vi "test-linear-system-loop-01.vi"() -> (3 "TEst Passed":bool)   [LabVIEW 2019]
uses:
  <vilib>/Rock Robotics/WPI/ThirdParty/JAS_Junk/TrajLib/Trajectory_Library.lvlib
  <vilib>/ptbypt/NI_PtbyPt.lvlib
  <vilib>/Rock Robotics/WPI/ThirdParty/JAS_Junk/TrajLib/DCMotor_GetVex775Pro.vi
  <vilib>/Analysis/Matrix/Datatypes/RealMatrix.ctl
  <vilib>/Analysis/Matrix/NI_Matrix.lvlib
  <vilib>/Rock Robotics/WPI/ThirdParty/JAS_Junk/TrajLib/TypeDef/LINEAR_QUADRATIC_REGULATOR.ctl
  <vilib>/Rock Robotics/WPI/ThirdParty/JAS_Junk/TrajLib/TypeDef/LINEAR_PLANT_INV_FF.ctl
  <vilib>/Rock Robotics/WPI/ThirdParty/JAS_Junk/TrajLib/TypeDef/LINEAR_SYSTEM.ctl
  <vilib>/Rock Robotics/WPI/ThirdParty/JAS_Junk/TrajLib/TypeDef/KALMAN_FILTER.ctl
  <vilib>/Rock Robotics/WPI/ThirdParty/JAS_Junk/TrajLib/TypeDef/LINEAR_SYSTEM_LOOP.ctl
panel:
  out "Waveform Graph":dbl[][](graph)
  out "Issue":bool
  out "Error":bool
  out "CorrError":bool
  out "out Linear System Loop":T1
  out "CalcYErr":bool
  out "LinSysLoopErr":bool
  out "LQRError":bool
  out "KalmanError":errorcluster
  out "Elev Sstem Err":bool
  # "<States,1>"
  # "<FUTURE --- CLAMP TYPE -- For now\nuse Normalize>"
  # "Steady State Gain  \n<States,Outputs>"
  # "State Estimate <Statess,1>"
  # "<States,States>"
  # "<States,Inputs>"
  # "<Outputs,States>"
  # "<Outputs,Inputs>"
  # "<States,1>"
  # "<Inputs,1>"
  # "<States,Inputs>"
  # "<States,States>"
  # "Ref State <States,1>"
  # "Comp and capped \noutput <Inputs,1>"
  # "Controller gain\n<Inputs,States>"
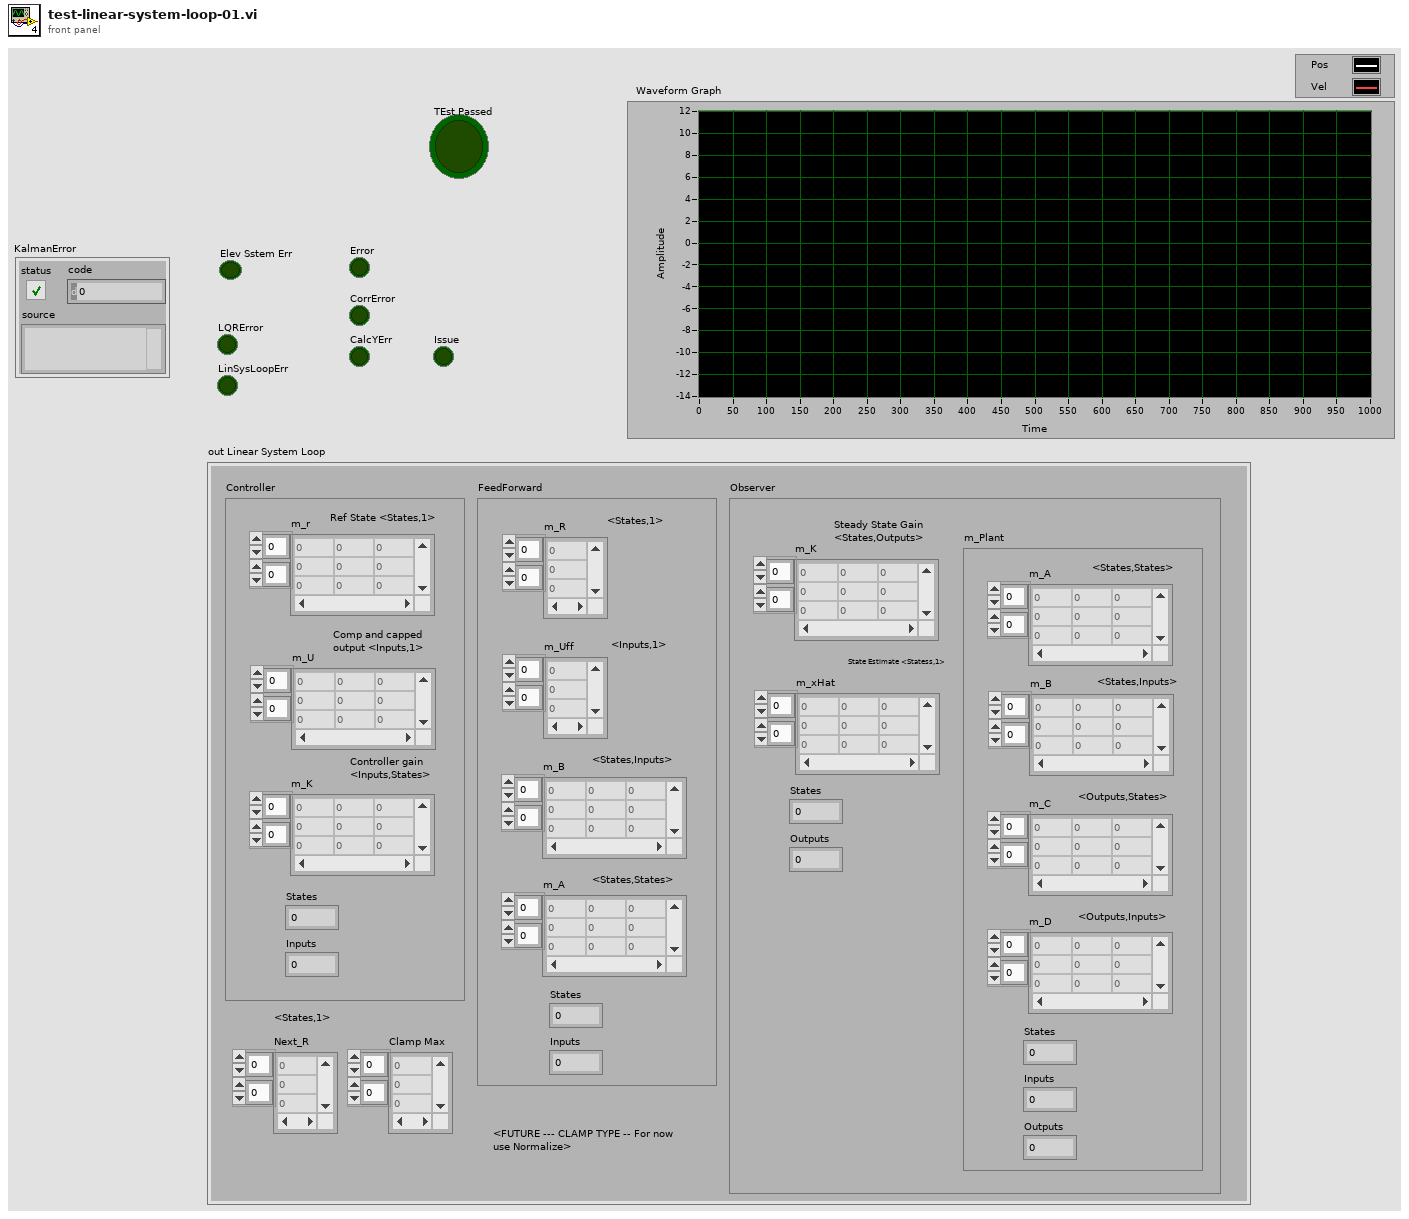
[diagram p1: front panel]
types:
  T1 = typedef "Trajectory_Library.lvlib/LINEAR_SYSTEM_LOOP.ctl" = cluster{"Controller":T2, "FeedForward":T4, "Observer":T5, "Next_R":T3, "Clamp Max":T3}
  T2 = typedef "Trajectory_Library.lvlib/LINEAR_QUADRATIC_REGULATOR.ctl" = cluster{"m_r":T3, "m_U":T3, "m_K":T3, "States":i32, "Inputs":i32}
  T3 = typedef "NI_Matrix.lvlib/RealMatrix.ctl" = dbl[][]
  T4 = typedef "Trajectory_Library.lvlib/LINEAR_PLANT_INV_FF.ctl" = cluster{"m_R":T3, "m_Uff":T3, "m_B":T3, "m_A":T3, "States":i32, "Inputs":i32}
  T5 = typedef "Trajectory_Library.lvlib/KALMAN_FILTER.ctl" = cluster{"m_K":T3, "m_xHat":T3, "States":i32, "Outputs":i32, "m_Plant":T6}
  T6 = typedef "Trajectory_Library.lvlib/LINEAR_SYSTEM.ctl" = cluster{"m_A":T3, "m_B":T3, "m_C":T3, "m_D":T3, "States":i32, "Inputs":i32, "Outputs":i32}
  T7 = typedef "Trajectory_Library.lvlib/DCMOTOR.CTL" = cluster{"nominalVoltage_Volts":dbl, "StallTorque_NM":dbl, "StallCurrent_Amps":dbl, "FreeCurrent_Amps":dbl, "FreeSpeed_RadPerSec":dbl, "R_Ohms":dbl, "KvINV_RadPerSecPerVolt":dbl, "Kt_NMPerAmp":dbl, "L_H":dbl, "Jr_KgM2":dbl}
  T8 = typedef "Trajectory_Library.lvlib/TRAPEZOID_PROFILE_CONSTRAINT.ctl" = cluster{"MaxVelocity":dbl, "MaxAcceleration":dbl}
  T9 = typedef "Trajectory_Library.lvlib/TRAPEZOID_PROFILE_STATE.ctl" = cluster{"Position":dbl, "Velocity":dbl}
  T10 = typedef "Trajectory_Library.lvlib/TRAPEZOID_PROFILE.ctl" = cluster{"EndAccel":dbl, "EndFullSpeed":dbl, "EndDecel":dbl, "Direction":i32, "Constraints":T8, "Initial":T9, "Goal":T9}
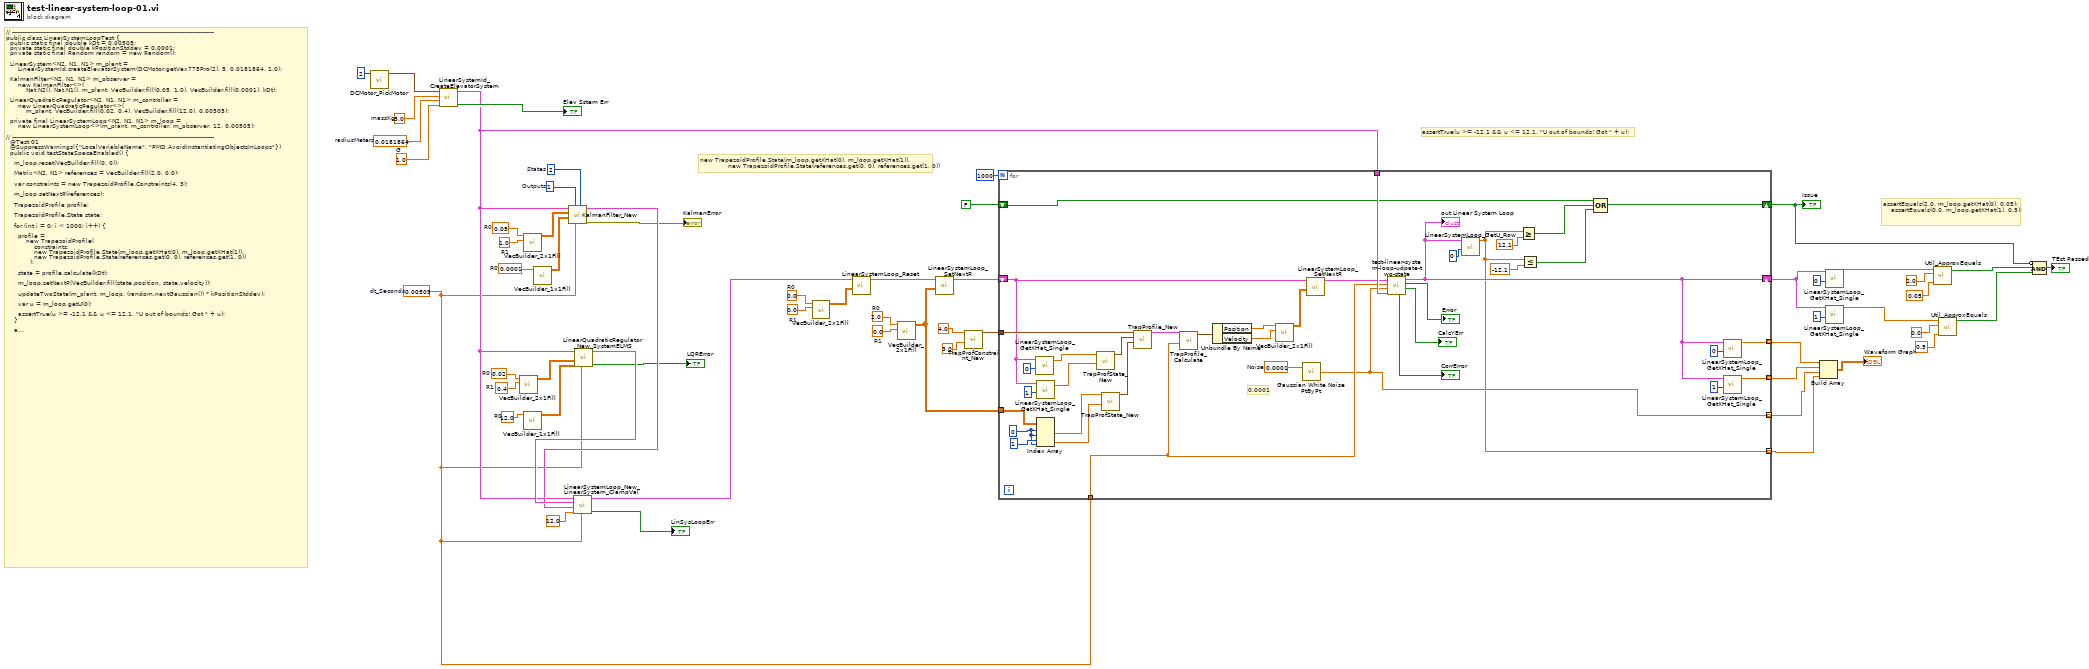
[diagram p0: block diagram]
diagram:
  w28 = 0.0  # R1
  w27 = 2.0  # R0
  w35 = 0.0  # R1
  w34 = 0.0  # R0
  w45 = 12.0  # R0
  w47 = 0.4  # R1
  w46 = 0.02  # R0
  w49 = 0.0001  # R0
  w51 = 1.0  # R1
  w50 = 0.05  # R0
  w52 = 1  # Outputs
  w21 = 0.00505  # dt_Seconds
  w53 = 2  # States
  w56 = 5.0  # massKg
  w57 = 0.0181864  # radiusMeters
  w58 = 1.0  # G
  # "assertEquals(2.0, m_loop.getXHat(0), 0.05);\n    assertEquals(0.0, m_loop.getXHat(1), 0.5);"
  # "assertTrue(u >= -12.1 && u <= 12.1, \"U out of bounds! Got \" + u);"
  # "new TrapezoidProfile.State(m_loop.getXHat(0), m_loop.getXHat(1)),\n              new TrapezoidProfile.State(references.get(0, 0), references.get(1, 0))"
  # "// -----------------------------------------------------------------------------------------------------\npublic class LinearSystemLoopTest {\n  public static final double kDt = 0.00505;\n  private static final double kPositionStddev = 0.0001;\n  private static final Random random = new Random();\n\n  LinearSystem<N2, N1, N1> m_plant =\n      LinearSystemId.createElevatorSystem(DCMotor.getVex775Pro(2), 5, 0.0181864, 1.0);\n\n  KalmanFilter<N2, N1, N1> m_observer =\n      new KalmanFilter<>(\n          Nat.N2(), Nat.N1(), m_plant, VecBuilder.fill(0.05, 1.0), VecBuilder.fill(0.0001), kDt);\n\n  LinearQuadraticRegulator<N2, N1, N1> m_controller =\n      new LinearQuadraticRegulator<>(\n          m_plant, VecBuilder.fill(0.02, 0.4), VecBuilder.fill(12.0), 0.00505);\n\n  private final LinearSystemLoop<N2, N1, N1> m_loop =\n      new LinearSystemLoop<>(m_plant, m_controller, m_observer, 12, 0.00505);\n\n// -----------------------------------------------------------------------------------------------------\n  @Test 01\n  @SuppressWarnings({\"LocalVariableName\", \"PMD.AvoidInstantiatingObjectsInLoops\"})\n  public void testStateSpaceEnabled() {\n\n    m_loop.reset(VecBuilder.fill(0, 0));\n\n    Matrix<N2, N1> references = VecBuilder.fill(2.0, 0.0);\n\n    var constraints = new TrapezoidProfile.Constraints(4, 3);\n\n    m_loop.setNextR(references);\n\n    TrapezoidProfile profile;\n\n    TrapezoidProfile.State state;\n\n    for (int i = 0; i < 1000; i++) {\n\n      profile =\n          new TrapezoidProfile(\n              constraints,\n              new TrapezoidProfile.State(m_loop.getXHat(0), m_loop.getXHat(1)),\n              new TrapezoidProfile.State(references.get(0, 0), references.get(1, 0))\n            );\n\n      state = profile.calculate(kDt);\n\n      m_loop.setNextR(VecBuilder.fill(state.position, state.velocity));\n\n      updateTwoState(m_plant, m_loop, (random.nextGaussian()) * kPositionStddev);\n\n      var u = m_loop.getU(0);\n\n      assertTrue(u >= -12.1 && u <= 12.1, \"U out of bounds! Got \" + u);\n    }\n\n    assertEquals(2.0, m_loop.getXHat(0), 0.05);\n    assertEquals(0.0, m_loop.getXHat(1), 0.5);\n  }"
  n1 = call-poly <vilib>:"DCMotor_PickMotor.vi"("Num Motors"=2) -> ("DCMOTOR"=w54:T7)  [unwired: 10 in]
  n2 = call <vilib>:"LinearSystemId_CreateElevatorSystem.vi"("G"=w58, "radiusMeters"=w57, "massKg"=w56, "DCMOTOR"=w54) -> ("Size Coerced"=→"Elev Sstem Err":bool, "Linearsystem"=w33:T6)  [unwired: 6 in]
  n3 = call <vilib>:"VecBuilder_2x1Fill.vi"("R1"=w47, "R0"=w46) -> ("output matrix"=w44:T3)  [unwired: 9 in]
  n4 = call <vilib>:"VecBuilder_1x1Fill.vi"("R0_C0"=w45) -> ("output matrix"=w43:T3)  [unwired: 10 in]
  n5 = call <vilib>:"VecBuilder_2x1Fill.vi"("R1"=w51, "R0"=w50) -> ("output matrix"=w48:T3)  [unwired: 9 in]
  n6 = call <vilib>:"VecBuilder_1x1Fill.vi"("R0_C0"=w49) -> ("output matrix"=w26:T3)  [unwired: 10 in]
  n7 = call <vilib>:"KalmanFilter_New.vi"("States"=w53, "dt_Seconds"=w21, "Outputs"=w52, "MeasurementStdDevs"=w26, "StateStdDevs"=w48, "Plant"=w33) -> ("Error"=→"KalmanError":errorcluster, "KalmanFilter"=w41:T5)  [unwired: 4 in]
  n8 = call <vilib>:"LinearQuadraticRegulator_New_SystemELMS.vi"("dt_Seconds"=w21, "Relms"=w43, "Qelms"=w44, "LINEARSYSTEM"=w33) -> ("Error"=→"LQRError":bool, "LinearQuadraticRegulator"=w42:T2)  [unwired: 6 in]
  n9 = call <vilib>:"LinearSystemLoop_New_LinearSystem_ClampVal.vi"("dT_Seconds"=w21, "Max_Voltage"=12.0, "Observer"=w41, "Controller"=w42, "Plant"=w33) -> ("Error"=→"LinSysLoopErr":bool, "Linear System Loop"=w32:T1)  [unwired: 5 in]
  n10 = call <vilib>:"VecBuilder_2x1Fill.vi"("R1"=w35, "R0"=w34) -> ("output matrix"=w31:T3)  [unwired: 9 in]
  n11 = call <vilib>:"LinearSystemLoop_Reset.vi"("initialState"=w31, "input inear System Loop"=w32) -> ("out Linear System Loop"=w30:T1)  [unwired: 8 in, 1 out]
  n12 = call <vilib>:"VecBuilder_2x1Fill.vi"("R1"=w28, "R0"=w27) -> ("output matrix"=w20:T3)  [unwired: 9 in]
  n13 = call <vilib>:"LinearSystemLoop_SetNextR.vi"("R"=w20, "input inear System Loop"=w30) -> ("out Linear System Loop"=w29:T1)  [unwired: 8 in, 1 out]
  n14 = call <vilib>:"TrapProfConstraint_New.vi"("Max Accel"=3.0, "Max Speed (M/S)"=4.0) -> ("TRAPEZOID_PROFILE_CONSTRAINT"=w22:T8)  [unwired: 9 in]
  n15 = for {
    N: 1000 -> [_]
    tunnel: w33 -> [w94]
    tunnel: w21 -> [w80]
    shift-right: [w63] -> w18
    shift-left: w29 -> [w76]
    tunnel: w22 -> [w93]
    tunnel: w20 -> [w84]
    shift-right: [w67] -> w6
    shift-left: FALSE -> [w66]
    tunnel: [w62] -> w9 mode=indexing
    tunnel: [w61] -> w8 mode=indexing
    tunnel: [w60] -> w2 mode=indexing
    tunnel: [w59] -> w1 mode=indexing
    w85 = 0 ("index (row)")
    w73 = 0.0001  # Noise
    # "0.0001"
    n16 = call <vilib>:"LinearSystemLoop_GetXHat_Single.vi"("Row"=0, "input inear System Loop"=w76) -> ("XHat"=w88:dbl)  [unwired: 9 in]
    n17 = call <vilib>:"LinearSystemLoop_GetXHat_Single.vi"("Row"=1, "input inear System Loop"=w76) -> ("XHat"=w87:dbl)  [unwired: 9 in]
    n18 = Index Array(array=w84, index (row) #1=w85, index (col) #1=w85, index (row) #2=1 ("index (row)"), index (col) #2=w85) -> (element #1=w83:dbl, element #2=w82:dbl)
    n19 = call <vilib>:"TrapProfState_New.vi"("Velocity"=w87, "Position"=w88) -> ("TRAPEZOID_PROFILE_STATE"=w92:T9)  [unwired: 9 in]
    n20 = call <vilib>:"TrapProfState_New.vi"("Velocity"=w82, "Position"=w83) -> ("TRAPEZOID_PROFILE_STATE"=w91:T9)  [unwired: 9 in]
    n21 = call <vilib>:"TrapProfile_New.vi"("Initial"=w91, "Goal"=w92, "Constraints"=w93) -> ("TRAPEZOID_PROFILE"=w81:T10)  [unwired: 8 in]
    n22 = call <vilib>:"TrapProfile_Calculate.vi"("Time"=w80, "TRAPEZOID_PROFILE"=w81) -> ("State"=w79:T9)  [unwired: 9 in]
    n23 = Unbundle By Name(w79) -> ("Position"=w78:dbl, "Velocity"=w77:dbl)
    n24 = call <vilib>:"VecBuilder_2x1Fill.vi"("R1"=w77, "R0"=w78) -> ("output matrix"=w74:T3)  [unwired: 9 in]
    n25 = call <vilib>:"Gaussian White Noise PtByPt.vi"("standard deviation"=w73) -> ("Gaussian white noise"=w60:dbl)  [unwired: 2 in]
    n26 = call <vilib>:"LinearSystemLoop_SetNextR.vi"("R"=w74, "input inear System Loop"=w76) -> ("out Linear System Loop"=w75:T1)  [unwired: 8 in, 1 out]
    n27 = call "test-linear-system-loop-udpate-two-state.vi"("Linearsystem"=w94, "Noise"=w60, "dt_Seconds"=w80, "Linear System Loop"=w75) -> ("CalcYErr"=→"CalcYErr":bool, "PredictError"=→"Error":bool, "out Linear System Loop"=w63:T1, "CorrectError"=→"CorrError":bool)  [unwired: 4 in]
    "out Linear System Loop" <- w63
    n28 = call <vilib>:"LinearSystemLoop_GetU_Row.vi"("Row"=0, "input inear System Loop"=w63) -> ("U"=w59:dbl)  [unwired: 9 in]
    n29 = Greater Or Equal?(x=w59, y=12.1) -> (x >= y?=w68:bool)
    n30 = Less Or Equal?(x=w59, y=-12.1) -> (x <= y?=w69:bool)
    n31 = Compound Arithmetic op=OR(w66, w68, w69) -> (w67:bool)
    n32 = call <vilib>:"LinearSystemLoop_GetXHat_Single.vi"("Row"=0, "input inear System Loop"=w63) -> ("XHat"=w62:dbl)  [unwired: 9 in]
    n33 = call <vilib>:"LinearSystemLoop_GetXHat_Single.vi"("Row"=1, "input inear System Loop"=w63) -> ("XHat"=w61:dbl)  [unwired: 9 in]
  }
  "Issue" <- w6
  n34 = Build Array(w9, w8, w2, w1) -> (→"Waveform Graph":dbl[][])
  n35 = call <vilib>:"LinearSystemLoop_GetXHat_Single.vi"("Row"=0, "input inear System Loop"=w18) -> ("XHat"=w13:dbl)  [unwired: 9 in]
  n36 = call <vilib>:"LinearSystemLoop_GetXHat_Single.vi"("Row"=1, "input inear System Loop"=w18) -> ("XHat"=w10:dbl)  [unwired: 9 in]
  n37 = call <vilib>:"Util_ApproxEquals.vi"("Tolerance"=0.05, "Value 2"=2.0, "Value 1"=w13) -> ("ApproxEquals"=w5:bool)  [unwired: 8 in]
  n38 = call <vilib>:"Util_ApproxEquals.vi"("Tolerance"=0.5, "Value 2"=0.0, "Value 1"=w10) -> ("ApproxEquals"=w4:bool)  [unwired: 8 in]
  n39 = Compound Arithmetic op=AND(invert w6, w5, w4) -> (→"TEst Passed":bool)
